vi "Validate XML.vi"() -> ()   [LabVIEW 2017]
uses:
  NationalInstruments.VeriStand.XMLReader
panel:
  out "error":string
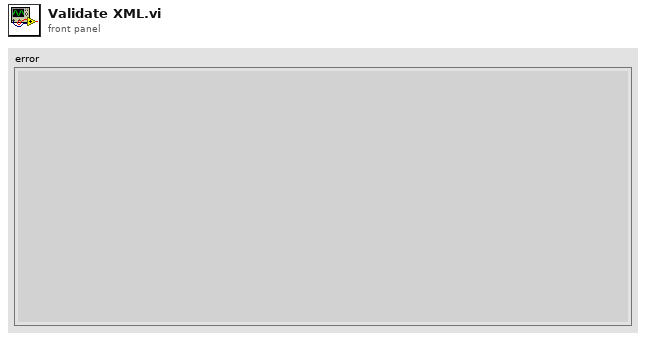
[diagram p1: front panel]
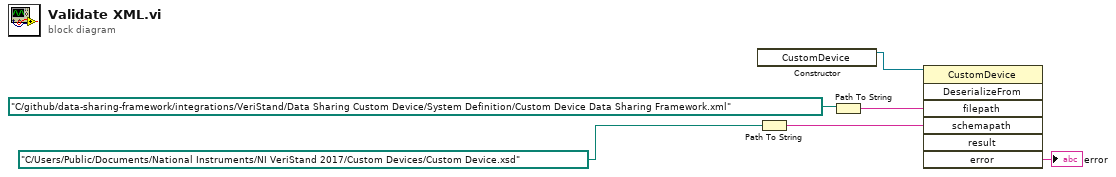
[diagram p0: block diagram]
diagram:
  n1 = constructor class="CustomDevice"() -> (reference out=w6:refnum<k24>)  [unwired: 3 in, 2 out]
  n2 = Path To String(path=path "C:/Users/Public/Documents/National Instruments/NI VeriStand 2017/Custom Devices/Custom Device.xsd" ("Path")) -> (string=w2:string)
  n3 = Path To String(path=path "C:/github/data-sharing-framework/integrations/VeriStand/Data Sharing Custom Device/System Definition/Custom Device Data Sharing Framework.xml" ("Path")) -> (string=w4:string)
  n4 = invoke class="CustomDevice" method="DeserializeFrom"(reference=w6, "filepath"=w4, "schemapath"=w2) -> ("error"=→"error":string)  [unwired: 4 in, 6 out]
